vi "Read Contestant Names.vi"(8 "error in (no error)":errorcluster, 11 "MC Prompt in":refnum<class "MC Prompt.lvclass">) -> (0 "error out":errorcluster, 2 "Contestant Names":string[](array[string]), 3 "MC Prompt out":refnum<class "MC Prompt.lvclass">)   [LabVIEW 2021, in "MC Prompt.lvlib" / "MC Prompt.lvclass"]
uses:
  MC Prompt.lvclass
  MC Prompt.lvclass/MC Prompt.ctl
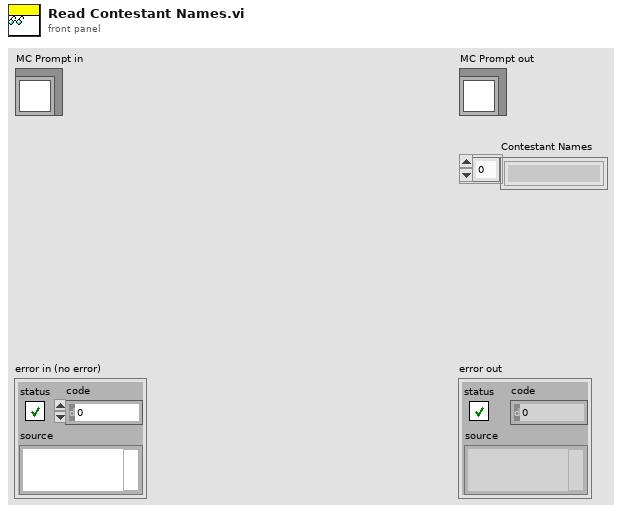
[diagram p1: front panel]
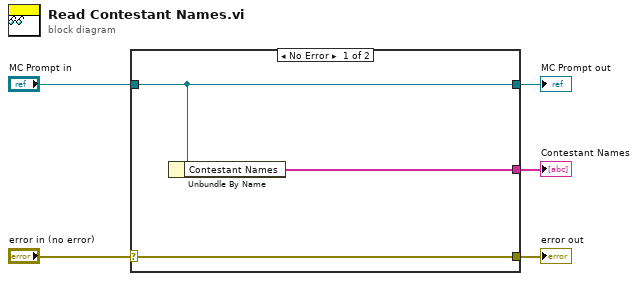
[diagram p0: block diagram]
diagram:
  n1 = case shown="No Error" "error in (no error)" {
    selector: "error in (no error)" -> [w8 w9]
    tunnel: [w8 w9] -> w4
    tunnel: [w7 w10] -> w2
    tunnel: "MC Prompt in" -> [w7 w10]
    tunnel: [w6 _] -> w1
    frame No Error {
      n2 = Unbundle By Name(w7) -> ("Contestant Names"=w6:string[])
    }
    frame Error {
    }
  }
  "error out" <- w4
  "MC Prompt out" <- w2
  "Contestant Names" <- w1
